vi "Test Run Tests.vi"(8 "error in":errorcluster) -> (0 "error out":errorcluster)   [LabVIEW 2020, in "UT_CICD.lvlib"]
doc: "Test call to run Unit, Integration, or End to End test VIs."
uses:
  UT_CICD.lvlib
  Test Types--enum.ctl
  8af4063a-b79b-4c67-82a3-c5fead23e19b.vi
  Source/CICD.lvlib
  <vilib>/addons/_JKI Toolkits/Caraya/classes/Test/Test.lvclass
  <vilib>/addons/_JKI Toolkits/Caraya/classes/Assert/Assert.lvclass
panel:
  out "Report paths":path[](array[path])
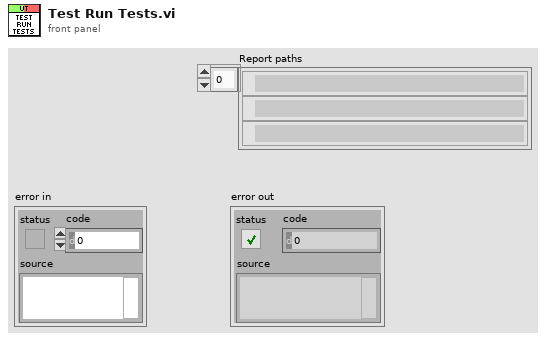
[diagram p1: front panel]
types:
  T1 = typedef "UT_CICD.lvlib/Test Types--enum.ctl" = enum16{"Unit", "Integration", "E2E"}
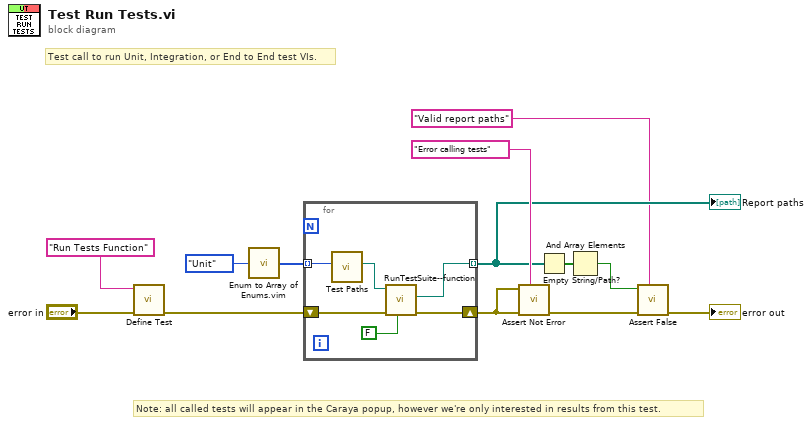
[diagram p0: block diagram]
diagram:
  # "Note: all called tests will appear in the Caraya popup, however we're only interested in results from this test."
  # "Test call to run Unit, Integration, or End to End test VIs."
  n1 = call <vilib>:"Define Test.vi"("error in (no error)"="error in", "Label (VI Title)"="Run Tests Function") -> ("error out"=w13:errorcluster)  [unwired: 8 in, 1 out]
  n2 = call "Enum to Array of Enums.vim"("enum"=Test_Types--enum."Unit" ("Test Type")) -> ("array of enums"=w9:T1[])
  n3 = for {
    tunnel: w9 -> [w17] mode=indexing
    tunnel: [w16] -> w5 mode=indexing
    shift-right: [w15] -> w7
    shift-left: w13 -> [w19]
    n4 = call "Test Paths.vi"("Test Type"=w17) -> ("Path"=w18:path)  [unwired: 10 in]
    n5 = call "RunTestSuite--function.vi"("Verbose (F)"=FALSE ("Interactive (F)"), "error in"=w19, "Test Suite (.vi)"=w18) -> ("error out"=w15:errorcluster, "Report Path"=w16:path)  [unwired: 6 in, 1 out]
  }
  "Report paths" <- w5
  n6 = call <vilib>:"Assert Not Error.vi"("Label"="Error calling tests", "error in (no error)"=w7, "Not Error?"=w7) -> ("error out"=w8:errorcluster)  [unwired: 7 in, 1 out]
  n7 = Empty String/Path?(string/path=w5) -> (empty?=w4:bool[])
  n8 = And Array Elements(Boolean array=w4) -> (logical AND=w2:bool)
  n9 = call <vilib>:"Assert False.vi"("Label"="Valid report paths", "error in (no error)"=w8, "False?"=w2) -> ("error out"=→"error out":errorcluster)  [unwired: 7 in, 1 out]
